vi "saveUniqueName.vi"(8 "error in (no error)":errorcluster, 10 "Check existence before modifying path":bool=TRUE, 11 "path":path) -> (0 "error out":errorcluster, 3 "unique path":path)   [LabVIEW 2011]
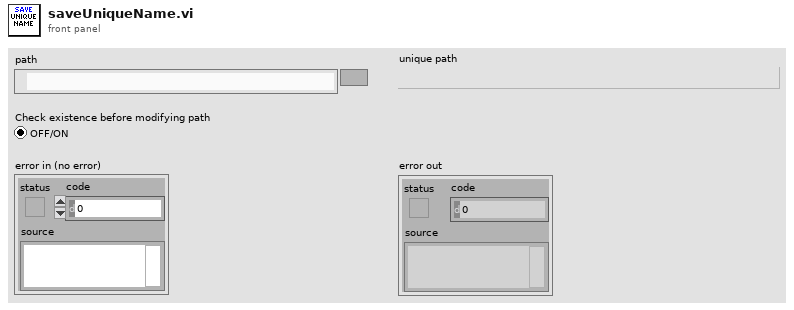
[diagram p1: front panel]
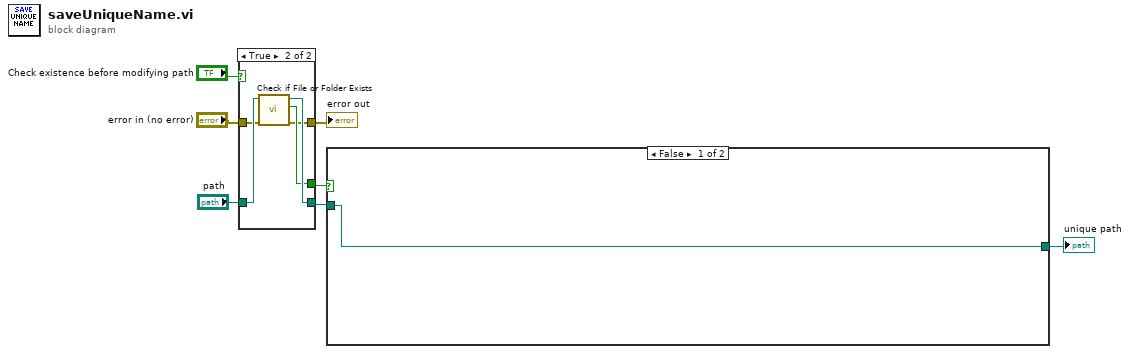
[diagram p0: block diagram]
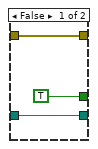
[diagram p2: hidden frame]
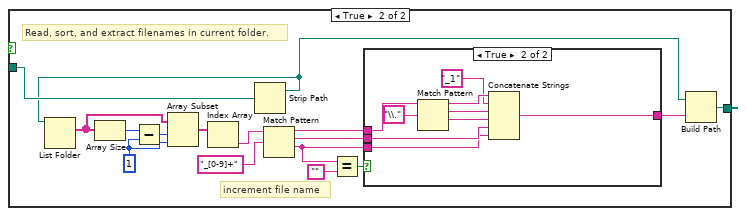
[diagram p3: hidden frame]
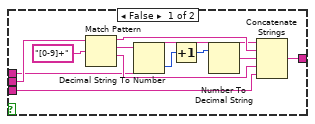
[diagram p4: hidden frame]
diagram:
  n1 = case shown="True" "Check existence before modifying path" {
    tunnel: "path" -> [w10 w15]
    tunnel: [w10 w14] -> w1
    tunnel: [TRUE ("file or folder exists?") w13] -> w4
    tunnel: "error in (no error)" -> [w8 w12]
    tunnel: [w8 w11] -> w6
    frame False {
    }
    frame True {
      n2 = call <vilib>:"Check if File or Folder Exists.vi"("error in (no error)"=w12, "path"=w15) -> ("error out"=w11:errorcluster, "file or folder exists?"=w13:bool, "dup path"=w14:path)  [unwired: 7 in]
    }
  }
  "error out" <- w6
  n3 = case shown="False" w4 {
    tunnel: w1 -> [w16 w19]
    tunnel: [w16 w28] -> w2
    frame False {
    }
    frame True {
      w20 = 1 ("length")
      # "Read, sort, and extract filenames in current folder."
      # "increment file name"
      n4 = Strip Path(path=w19) -> (stripped path=w17:path)  [unwired: 1 out]
      n5 = List Folder(path=w17) -> (filenames=w21:string[])  [unwired: 3 in, 3 out]
      n6 = Array Size(array=w21) -> (size(s)=w22:i32)
      n7 = Subtract(x=w22, y=w20) -> (x-y=w23:i32)
      n8 = Array Subset(array=w21, index=w23, length=w20) -> (w24:string[])
      n9 = Index Array(array=w24) -> (element=w18:string)  [unwired: 1 in]
      n10 = Match Pattern(string=w18, regular expression="_[0-9]+") -> (before substring=w29:string, match substring=w26:string, after substring=w25:string)  [unwired: 1 in, 1 out]
      n11 = Equal?(x=w25, y="") -> (x = y?=w30:bool)
      n12 = case shown="True" w30 {
        tunnel: w29 -> [w33 w52]
        tunnel: [w37 w44] -> w27
        tunnel: w26 -> [w43 w46]
        tunnel: w25 -> [w34 w45]
        frame False {
          n13 = Match Pattern(string=w43, regular expression="[0-9]+") -> (before substring=w36:string, match substring=w41:string, after substring=w35:string)  [unwired: 1 in, 1 out]
          n14 = Decimal String To Number(string=w41) -> (number=w40:i32)  [unwired: 2 in, 1 out]
          n15 = Increment(x=w40) -> (x+1=w39:i32)
          n16 = Number To Decimal String(number=w39) -> (decimal integer string=w38:string)  [unwired: 1 in]
          n17 = Concatenate Strings(w33, w36, w38, w35, w34) -> (w37:string)
        }
        frame True {
          n18 = Match Pattern(string=w52, regular expression="\\.") -> (before substring=w50:string, match substring=w48:string, after substring=w47:string)  [unwired: 1 in, 1 out]
          n19 = Concatenate Strings(w50, "_1" ("string"), w48, w47, w46, w45) -> (w44:string)
        }
      }
      n20 = Build Path(base path=w17, name or relative path=w27) -> (appended path=w28:path)
    }
  }
  "unique path" <- w2
